vi "1 byte read.vi"(3 "Min time SCL low (uSec)":u32, 4 "Min Time SCL high (uSec)":u32) -> (2 "Data bit array":bool[](array[boolean]))   [LabVIEW 2013]
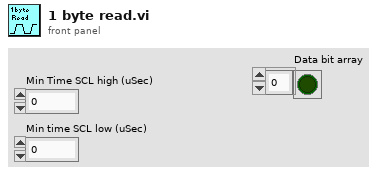
[diagram p1: front panel]
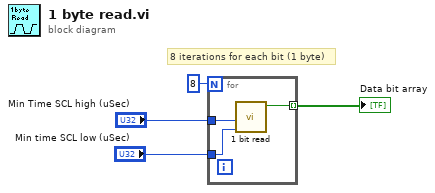
[diagram p0: block diagram]
diagram:
  # "8 iterations for each bit (1 byte)"
  n1 = for {
    N: 8 -> [_]
    tunnel: "Min Time SCL high (uSec)" -> [w7]
    tunnel: "Min time SCL low (uSec)" -> [w6]
    tunnel: [w5] -> w1 mode=indexing
    n2 = call "1 bit read.vi"("Min time SCL low (uSec)"=w6, "Min Time SCL high (uSec)"=w7) -> ("Data bit"=w5:bool)  [unwired: 5 in]
  }
  "Data bit array" <- w1
